vi "acquire_single.vi"(8 "error in (no error)":errorcluster, 10 "Frequency (Hz)":dbl, 11 "Resonance Curve in":refnum<class "Resonance Curve.lvclass">) -> (0 "error out":errorcluster, 1 "Phase (rad)":dbl, 2 "Amplitude (V rms)":dbl, 3 "Resonance Curve out":refnum<class "Resonance Curve.lvclass">)   [LabVIEW 2020, in "Resonance Curve.lvclass"]
uses:
  Resonance Curve.lvclass
  Resonance Curve.lvclass/Resonance Curve.ctl
  <vilib>/Analysis/baseanly.llb/Mean (DBL).vi
  Function Generator/Function Generator.lvclass
  Lock-In Amplifier/Lock-In Amplifier.lvclass
  <vilib>/Analysis/NI_AALBase.lvlib
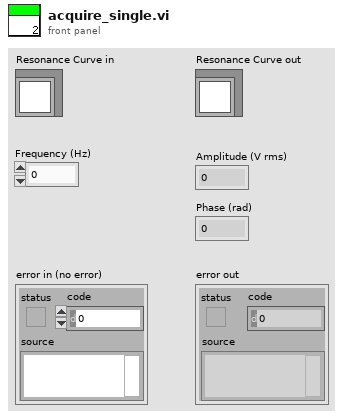
[diagram p1: front panel]
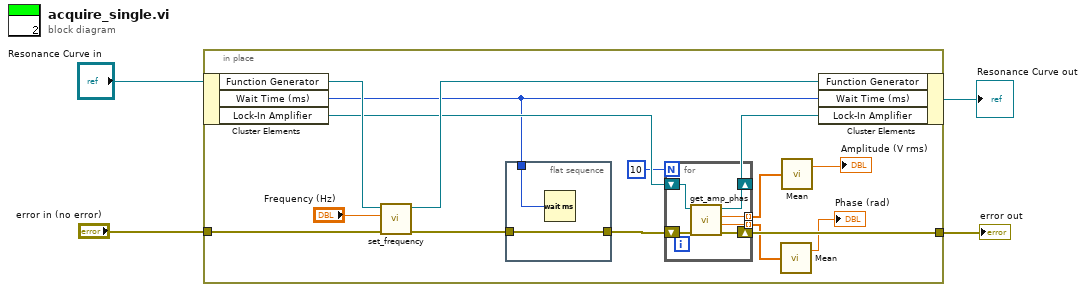
[diagram p0: block diagram]
diagram:
  n1 = in-place {
    in-place-border: "error in (no error)" -> [w16]
    in-place-border: [w10] -> w2
    n2 = in-place-cluster #1("Resonance Curve in") -> ("Function Generator"=w18:refnum<class "Function Generator.lvclass">, "Wait Time (ms)"=w12:u32, "Lock-In Amplifier"=w13:refnum<class "Lock-In Amplifier.lvclass">)
    n3 = call-dynamic "set_frequency.vi"("error in (no error)"=w16, "Frequency"="Frequency (Hz)", "Function Generator in"=w18) -> ("error out"=w15:errorcluster, "Function Generator out"=w17:refnum<class "Function Generator.lvclass">)  [unwired: 7 in]
    n4 = flat-sequence {
      tunnel: w12 -> [w27]
      tunnel: w15 -> [w26]
      tunnel: [w26] -> w14
      frame #0 {
        n5 = Wait (ms)(milliseconds to wait=w27) -> ()  [unwired: 1 out]
      }
    }
    n6 = for {
      N: 10 -> [_]
      tunnel: [w21] -> w9 mode=indexing
      tunnel: [w20] -> w7 mode=indexing
      shift-right: [w22] -> w10
      shift-left: w14 -> [w25]
      shift-right: [w23] -> w11
      shift-left: w13 -> [w24]
      n7 = call-dynamic "get_amp_phas.vi"("error in (no error)"=w25, "Lock-In Amplifier in"=w24) -> ("error out"=w22:errorcluster, "Phase (rad)"=w20:dbl, "Amplitude (V rms)"=w21:dbl, "Lock-In Amplifier out"=w23:refnum<class "Lock-In Amplifier.lvclass">)  [unwired: 6 in]
    }
    n8 = call-poly <vilib>:"Mean.vi"("X"=w7) -> ("mean"=→"Phase (rad)":dbl)  [unwired: 1 out]
    n9 = call-poly <vilib>:"Mean.vi"("X"=w9) -> ("mean"=→"Amplitude (V rms)":dbl)  [unwired: 1 out]
    n10 = in-place-cluster #1("Function Generator"=w17, "Wait Time (ms)"=w12, "Lock-In Amplifier"=w11) -> (→"Resonance Curve out":refnum<class "Resonance Curve.lvclass">)
  }
  "error out" <- w2
